vi "2_1_PatchCore_Inference(Image)(Batch).vi"() -> ()   [LabVIEW 2020]
uses:
  PatchCore_AddOn/API/Controls/Heatmap_Config.ctl
  PatchCore_AddOn/API/Controls/ColorMap.ctl
  PatchCore_AddOn/API/Controls/MinMax.ctl
  PatchCore_AddOn/API/Controls/Feature_Scorer_Params.ctl
  PatchCore_AddOn/API/Controls/Gaussian_Blur.ctl
  PatchCore_AddOn/API/Controls/NNPC_Init_Custom_NN_CFG.ctl
  <vilib>/Ngene/Deep Learning Toolkit/Toolkit/NN_Data/API/NN_Dims(C,H,W).ctl
  PatchCore_AddOn/API/Controls/NNPC_Device.ctl
  <vilib>/Ngene/Deep Learning Toolkit/Toolkit/NN_Network/Controls/NN_Device.ctl
  PatchCore_AddOn/API/Controls/NNPC_Trained_Model_Paths.ctl
  PatchCore_AddOn/API/Controls/NN_Paths.ctl
  <vilib>/Utility/miscctls.llb/LVMinMaxIncTypeDef.ctl
  subVIs/Dataset_Reader/Controls/ImRead_PreProcessing_Options.ctl
  PatchCore_AddOn/Low_Level/Controls/Normalization_Type.ctl
  <vilib>/Analysis/baseanly.llb/Mean (DBL).vi
  PatchCore_AddOn/API/NNPC_Predict/NNPC_Predict(Batch).vi
  PatchCore_AddOn/PatchCore_AddOn.lvlib
  <vilib>/ptbypt/NI_PtbyPt.lvlib
  <vilib>/Analysis/NI_AALBase.lvlib
  <vilib>/Ngene/Deep Learning Toolkit/Toolkit/Deep_Learning_Toolkit_by_Ngene.lvlib
panel:
  in  "NNFE PatchCore Paths":T1={"NNFE_Paths"={"CFG"=path "D:/PatchCore/__24_12_11__22_07_40/wrn_50_2_timm_NNFE__24_12_11__22_07_40.cfg", "BIN"=path "D:/PatchCore/__24_12_11__22_07_40/wrn_50_2_timm_NNFE__24_12_11__22_07_40.bin"}, "PatchCore_Paths"={"CFG"=path "D:/PatchCore/__24_12_11__22_07_40/wrn_50_2_timm_Patchcore__24_12_11__22_07_40.cfg", "BIN"=path "D:/PatchCore/__24_12_11__22_07_40/wrn_50_2_timm_MemBank__PS3_RP296_SR0.1_Size16.4k__24_12_11__22_07_40.bin"}}
  in  "Device_Config.":T3={"Device"=enum."GPU", "GPU Id"=0}
  in  "Eval_Stats_File_Path":path=path "D:/PatchCore/__24_12_11__22_07_40/PatchCore_Eval_Stats__24_12_11__22_13_40.cfg"
  in  "NNFE_Custom_CFG":T5={"Input3D_Custom_Dims"={"C"=-1, "H"=-1, "W"=-1}, "mBatch"=8}
  in  "Ground_Truth_Folder_Path":path=path "D:/MVTec/bottle/ground_truth"
  in  "Test_Dataset_Folder_Path":path=path "D:/MVTec/bottle/test"
  in  "Batch_idx":u32 max=74
  in  "Pixel_Thrshld(Custom)":sgl=-1.0 format="%_5g"
  out "Img_Score":sgl=22.713667
  out "Anomaly Detection Results":T7(plugin-control)
  out "Anomaly?":bool
  in  "Stop":bool
  out "Pixel_Thrshld (Eval)":sgl=25.5661
  out "dT_ImRead":dbl=0.02234118052628889 format="%#_4ps"
  out "Image_File_Path":path=path "D:/MVTec/bottle/test/good/000.png"
  out "Pixel_Score(Max)":sgl=27.324837
  out "Pixel_Score(Min)":sgl=2.317538
  out "dT_Predict(Batch)":dbl=0.0410997536842938 format="%#_3ps"
  in  "Feature_Scorer_Params":T8={"Nearest_Neihbours"=1, "Calculate Anomaly Map"=TRUE, "Gaussian_Blur"={"Kernel_Size"=33, "sigma"=4.0}}
  in  "Report_Image_Dims":cluster{"X Resolution":i32, "Y Resolution":i32}={"X Resolution"=224, "Y Resolution"=224}
  in  "Heatmap_Config":T10={"ColorMap_Type"=enum."Jet", "Alpha"=0.4, "Heatmap Range"={"Min"=-1.0, "Max"=-1.0}} {"Heatmap Range"."Min" format="%#_5g"}
  in  "Image_Thrshld(Custom)":sgl=-1.0 format="%_5g"
  out "Image_Thrshld (Eval)":sgl=30.7657
  in  "Image_idx":u32 max=7
  out "Batch Image File Paths":path[](array[path])=[path "D:/MVTec/bottle/test/good/000.png", path "D:/MVTec/bottle/test/good/001.png", path "D:/MVTec/bottle/test/good/002.png", path "D:/MVTec/bottle/test/good/003.png", path "D:/MVTec/bottle/test/good/004.png", path "D:/MVTec/bottle/test/good/005.png", path "D:/MVTec/bottle/test/good/006.png", path "D:/MVTec/bottle/test/good/007.png"]
  out "Anomaly?(Batch)":bool[](array[boolean])
  out "Img_Scores(Batch)":sgl[](array[numeric])=[22.713667, 29.501556, 24.734844, 22.781378, 22.935541, 22.427269, 25.48138, 22.724445]
  out "dT_Predict(perImg)":dbl=0.005137469210536725 format="%#_3ps"
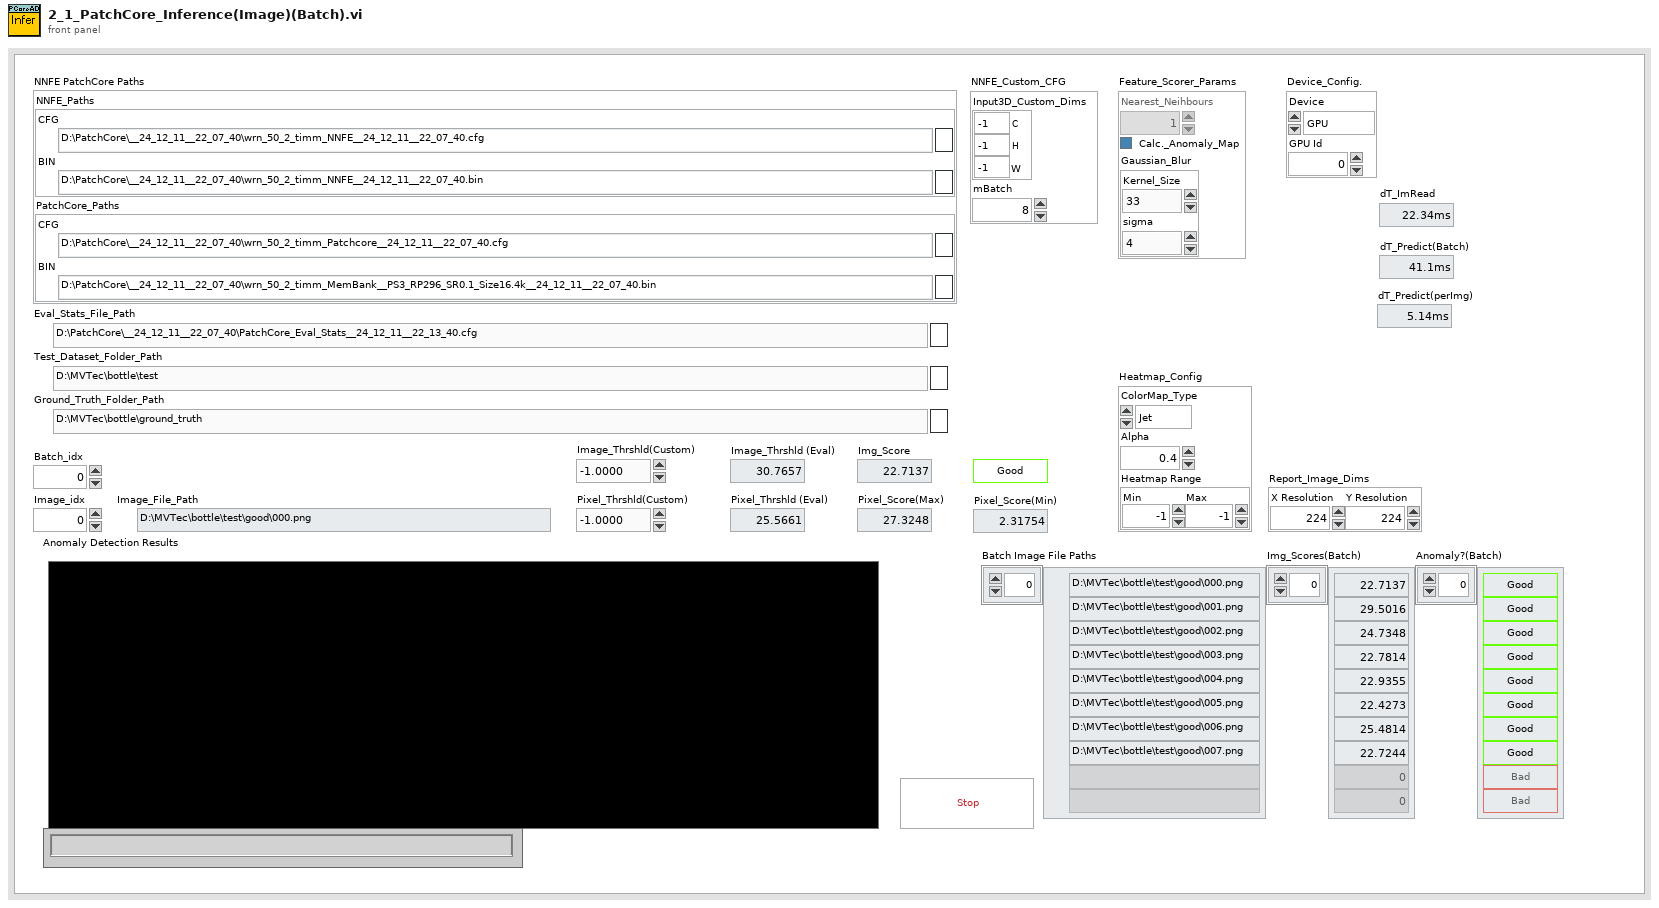
[diagram p1: front panel]
types:
  T1 = typedef "PatchCore_AddOn.lvlib/NNPC_Trained_Model_Paths.ctl" = cluster{"NNFE_Paths":T2, "PatchCore_Paths":T2}
  T2 = typedef "PatchCore_AddOn.lvlib/NN_Paths.ctl" = cluster{"CFG":path, "BIN":path}
  T3 = typedef "PatchCore_AddOn.lvlib/NNPC_Device.ctl" = cluster{"Device":T4, "GPU Id":i32}
  T4 = typedef "Deep_Learning_Toolkit_by_Ngene.lvlib/NN_Device.ctl" = enum16{"CPU", "GPU"}
  T5 = typedef "PatchCore_AddOn.lvlib/NNPC_Init_Custom_NN_CFG.ctl" = cluster{"Input3D_Custom_Dims":T6, "mBatch":i32}
  T6 = typedef "Deep_Learning_Toolkit_by_Ngene.lvlib/NN_Dims(C,H,W).ctl" = cluster{"C":i32, "H":i32, "W":i32}
  T7 = typedef "IMAQ Image.ctl" = refnum<image>
  T8 = typedef "PatchCore_AddOn.lvlib/Feature_Scorer_Params.ctl" = cluster{"Nearest_Neihbours":i32, "Calculate Anomaly Map":bool, "Gaussian_Blur":T9}
  T9 = typedef "PatchCore_AddOn.lvlib/Gaussian_Blur.ctl" = cluster{"Kernel_Size":i32, "sigma":sgl}
  T10 = typedef "PatchCore_AddOn.lvlib/Heatmap_Config.ctl" = cluster{"ColorMap_Type":T11, "Alpha":sgl, "Heatmap Range":T12}
  T11 = typedef "PatchCore_AddOn.lvlib/ColorMap.ctl" = enum16{"Jet", "Perula", "Inferno", "Plasma", "Viridis"}
  T12 = typedef "PatchCore_AddOn.lvlib/MinMax.ctl" = cluster{"Min":sgl, "Max":sgl}
  T13 = typedef "LVMinMaxIncTypeDef.ctl" = cluster{"Minimum":dbl, "Maximum":dbl, "Increment":dbl}
  T14 = typedef "PatchCore_AddOn.lvlib/NNPC_Instance.ctl" = cluster{"Dataset_Stats":T15, "NN":T17, "Device_Config.":T3, "PatchCore_Init_CFG":T32, "Coreset Params":T34, "MemBank_Data":T36}
  T15 = typedef "PatchCore_AddOn.lvlib/NNPC_DS_Stats.ctl" = cluster{"means":T16, "vars":T16, "DS_Size":i32}
  T16 = typedef "PatchCore_AddOn.lvlib/Image_Stats_RGB.ctl" = cluster{"R":sgl, "G":sgl, "B":sgl}
  T17 = typedef "Deep_Learning_Toolkit_by_Ngene.lvlib/NN.ctl" = cluster{"Name":string, "No of Layers":i32, "mBatch":i32, "Layers":T18[], "Dimty":T19, "Dims_In":T6, "Dims_Out":T6, "Working_Dir":path, "Train?":bool, "Train_Params":T20, "LR_Update_Policy":T23, "Session Data":T25, "Ground_truth":T26, "NNg_hdls":T27, "NN_Device":T4, "GPU Id":i32, "Labels":string[], "Receptive Field":T28[], "Loss_Type":T29, "Loss_Cfg_Prms":variant, "NNG_WS":T30}
  T18 = typedef "Deep_Learning_Toolkit_by_Ngene.lvlib/NN_Layer_ref.ctl" = refnum<data-value>
  T19 = typedef "Deep_Learning_Toolkit_by_Ngene.lvlib/NN_In_Out_Dim-ty.ctl" = enum8{"In1D_Out1D", "In3D_Out1D", "In3D_Out3D", "In3D_OutBBox"}
  T20 = typedef "Deep_Learning_Toolkit_by_Ngene.lvlib/NN_Train_Params.ctl" = cluster{"Optimizer":T21, "Beta_1":sgl, "Beta_2":sgl, "Weight Decay(L1)":sgl, "Weight Decay(L2)":sgl, "Data_Sampling":T22}
  T21 = typedef "Deep_Learning_Toolkit_by_Ngene.lvlib/NN_Train_Optimizer.ctl" = enum16{"SGD", "Adam", "Adagrad", "Adadelta", "RMSProp", "Nesterov"}
  T22 = typedef "Deep_Learning_Toolkit_by_Ngene.lvlib/NN_Train_Data_Sampling.ctl" = enum16{"Random", "Sequential"}
  T23 = typedef "Deep_Learning_Toolkit_by_Ngene.lvlib/NN_LR_Policy_Cfg.ctl" = cluster{"Policy_Type":T24, "LR0":dbl, "k":sgl, "WarmUp_Policy":enum16{"Step", "Ramp"}, "WarmUp_Iter":i32, "WarmUp_Ratio":sgl}
  T24 = typedef "Deep_Learning_Toolkit_by_Ngene.lvlib/NN_LR_Policy_Type.ctl" = enum16{"Manual", "Step", "Exp", "1/t"}
  T25 = typedef "Deep_Learning_Toolkit_by_Ngene.lvlib/NN_Train_Session_Data.ctl" = cluster{"Epochs":sgl, "Tot_Iter":i32, "LR":sgl, "LR_iter":i32}
  T26 = typedef "Deep_Learning_Toolkit_by_Ngene.lvlib/NN_Ground_truth.ctl" = cluster{"Y":variant}
  T27 = typedef "Deep_Learning_Toolkit_by_Ngene.lvlib/nng_cuda_handles.ctl" = cluster{"cudnn":u64, "cublas":u64, "stream":u64, "curand":u64}
  T28 = typedef "Deep_Learning_Toolkit_by_Ngene.lvlib/NN_Dims(V,H).ctl" = cluster{"V":i32, "H":i32}
  T29 = typedef "Deep_Learning_Toolkit_by_Ngene.lvlib/NN_Loss_Type.ctl" = enum16{"None", "MSE", "CrossEntropy", "YOLO_v2", "YOLO_v4"}
  T30 = typedef "Deep_Learning_Toolkit_by_Ngene.lvlib/NNG_WS.ctl" = cluster{"NNG_WS_Mem":T31, "Max_WS_Size":i64}
  T31 = typedef "Deep_Learning_Toolkit_by_Ngene.lvlib/NNg_WS_Mem_DVR.ctl" = refnum<data-value>
  T32 = typedef "PatchCore_AddOn.lvlib/NNPC_Init_CFG.ctl" = cluster{"BackBone":T33, "Out_Layers_Names":string[], "Patch_Size":u32}
  T33 = typedef "PatchCore_AddOn.lvlib/NNPC_BackBone_Selector.ctl" = enum16{"WRN_50_2_L2L3"}
  T34 = typedef "PatchCore_AddOn.lvlib/NNPC_Coreset_Params.ctl" = cluster{"Name":string, "Sampling_Ratio":sgl, "Startd_idx":i32, "Random_Proj?":bool, "Rnd. Proj. Params":T35}
  T35 = typedef "PatchCore_AddOn.lvlib/NNPC_Random_Projection_CFG.ctl" = cluster{"Proj._Dim.":i32, "Epsilon":sgl, "Seed":i32}
  T36 = typedef "PatchCore_AddOn.lvlib/MemBank_and_Norm_Variants.ctl" = cluster{"MemBank":variant, "MemBank Norm":variant}
  T37 = typedef "PatchCore_AddOn.lvlib/Eval_Results.ctl" = cluster{"Scores(Good)":T12, "Scores(Bad)":T12, "F1_Max":sgl, "Thrshld(F1_Max)":sgl, "IoU_Max":sgl, "Thrshld(IoU_Max)":sgl, "AUROC":sgl, "Prec.(F1_Max)":sgl, "Recall(F1_Max)":sgl, "FPR(F1_Max)":sgl, "FNR(F1_Max)":sgl}
  T38 = typedef "ImRead_PreProcessing_Options.ctl" = cluster{"Image Type":T39, "Normalization Type":T40, "Interpolation Type":u32}
  T39 = typedef "Image Type" = u32
  T40 = typedef "PatchCore_AddOn.lvlib/Normalization_Type.ctl" = enum16{"Standardize(DS_Stats)", "Standardize(Image_Stats)"}
  T41 = typedef "PatchCore_AddOn.lvlib/Anomaly_Detection_Results_Imgs.ctl" = cluster{"Image":T7, "Ground Truth":T7, "Predicted Heat Map":T7, "Predicted Mask":T7, "Segmentation":T7}
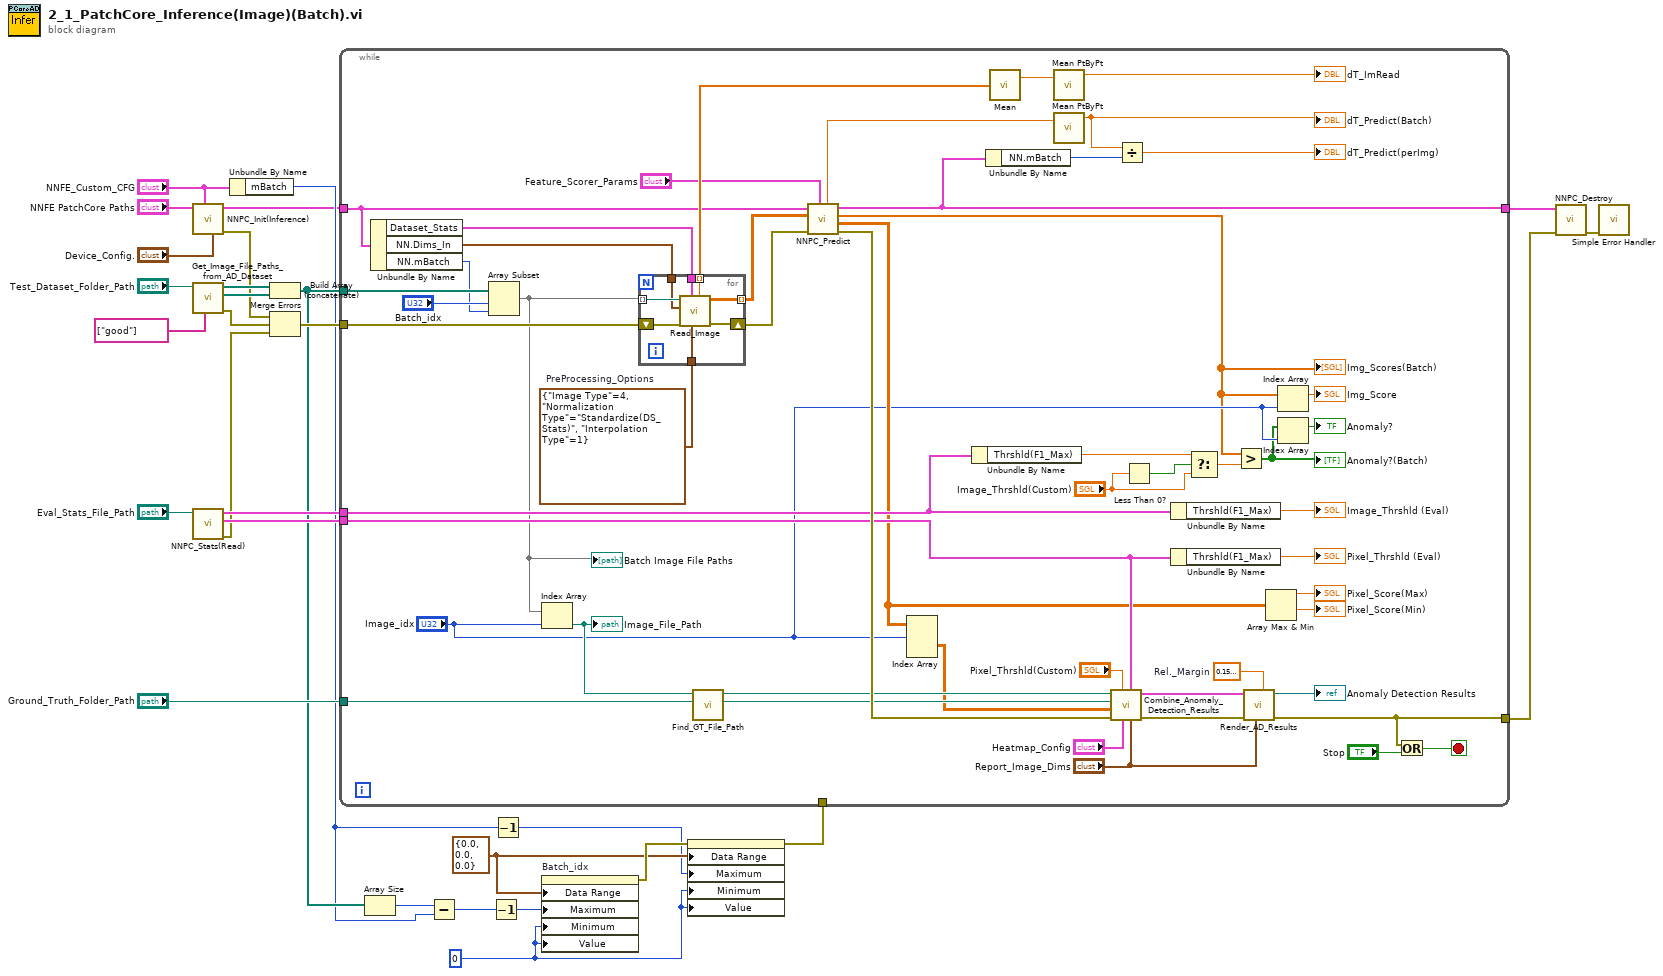
[diagram p0: block diagram]
diagram:
  w11 = T13 {"Minimum"=0.0, "Maximum"=0.0, "Increment"=0.0} ("Data Entry Limits")
  w9 = u32 0 ("Data Entry Limits:Minimum")
  n1 = call "NNPC_Init(Inference).vi"("Device_Config."="Device_Config.", "NNFE_Custom_CFG"="NNFE_Custom_CFG", "NNFE PatchCore Paths"="NNFE PatchCore Paths") -> ("error out"=w2:errorcluster, "PCore_Instance out"=w5:T14)  [unwired: 7 in]
  n2 = call "Get_Image_File_Paths_from_AD_Dataset.vi"("Good Folder Names"=string[] ["good"] ("Good Folder Name"), "Dataset Folder"="Test_Dataset_Folder_Path") -> ("error out"=w18:errorcluster, "Bad Dataset Files"=w14:path[], "Good Dataset Files"=w13:path[])  [unwired: 7 in]
  n3 = call "NNPC_Stats(Read).vi"("CFG file path"="Eval_Stats_File_Path") -> ("error out"=w22:errorcluster, "Pixel Results"=w23:T37, "Image Results"=w24:T37)  [unwired: 8 in]
  n4 = Unbundle By Name("NNFE_Custom_CFG") -> ("mBatch"=w7:i32)
  n5 = Build Array (concatenate)(w13, w14) -> (w19:path[])
  n6 = Merge Errors(w2, w18, w22) -> (w25:errorcluster)
  n7 = Array Size(array=w19) -> (size(s)=w29:i32)
  n8 = Subtract(x=w29, y=w7) -> (x-y=w8:i32)
  n9 = Decrement(x=w8) -> (x-1=w28:i32)
  n10 = Decrement(x=w7) -> (x-1=w10:i32)
  n11 = property on="Batch_idx" class="DigNum (strict)"("Data Range"=w11, "Maximum"=w28, "Minimum"=w9, "Value"=w9) -> (error out=w12:errorcluster)  [unwired: 2 in, 1 out]
  n12 = property on="Image_idx" class="DigNum (strict)"(error in=w12, "Data Range"=w11, "Maximum"=w10, "Minimum"=w9, "Value"=w9) -> (error out=w6:errorcluster)  [unwired: 1 in, 1 out]
  n13 = while {
    tunnel: w19 -> [w81]
    tunnel: w5 -> [w61]
    tunnel: [w33] -> w16
    tunnel: w24 -> [w55]
    tunnel: w23 -> [w54]
    tunnel: w25 -> [w80]
    tunnel: [w30] -> w17
    tunnel: "Ground_Truth_Folder_Path" -> [w64]
    tunnel: w6 -> [_]
    stop <- w31 stop-if-true
    w73 = sgl 0.15  # Rel._Margin
    w50 = T38 {"Image Type"=4, "Normalization Type"=enum."Standardize(DS_Stats)", "Interpolation Type"=1}  # PreProcessing_Options
    n14 = Unbundle By Name(w61) -> ("Dataset_Stats"=w52:T15, "NN.Dims_In"=w51:T6, "NN.mBatch"=w46:i32)
    n15 = Array Subset(array=w81, index="Batch_idx", length=w46) -> (w47:path[])
    "Batch Image File Paths" <- w47
    n16 = Index Array(array=w47, index="Image_idx") -> (element=w48:path)
    "Image_File_Path" <- w48
    n17 = for {
      tunnel: [w88] -> w67 mode=indexing
      tunnel: w47 -> [w87] mode=indexing
      tunnel: [w86] -> w38 mode=indexing
      tunnel: w52 -> [w84]
      tunnel: w51 -> [w83]
      tunnel: w50 -> [w82]
      shift-right: [w85] -> w53
      shift-left: w80 -> [w89]
      n18 = call "Read_Image.vi"("PreProcessing_Options"=w82, "Dataset_Stats"=w84, "error in"=w89, "Target_Dims"=w83, "Img Path"=w87) -> ("error out"=w85:errorcluster, "Image Out"=w86:sgl[][][], "dT_Img_Read"=w88:dbl)  [unwired: 4 in]
    }
    n19 = call "Find_GT_File_Path.vi"("GT Mask Folder Path"=w64, "Image File Path"=w48) -> ("GT File Path"=w65:path, "Image File Path out"=w66:path)  [unwired: 8 in]
    n20 = call-poly "NNPC_Predict.vi"("Feature Scorer Params"="Feature_Scorer_Params", "error in (no error)"=w53, "Image(Batch)"=w38, "PCore_Instance in"=w61) -> ("error out"=w78:errorcluster, "anomaly maps"=w44:sgl[][][], "pred scores"=w39:sgl[], "PCore_Instance out"=w33:T14, "dT_Predict"=w60:dbl)  [unwired: 3 in]
    "Img_Scores(Batch)" <- w39
    n21 = Index Array(array=w44, index (dim 0)="Image_idx") -> (element=w45:sgl[][])  [unwired: 2 in]
    n22 = Unbundle By Name(w55) -> ("Thrshld(F1_Max)"=w69:sgl)
    n23 = Unbundle By Name(w33) -> ("NN.mBatch"=w32:i32)
    n24 = call-poly <vilib>:"Mean.vi"("X"=w67) -> ("mean"=w37:dbl)  [unwired: 1 out]
    n25 = call <vilib>:"Mean PtByPt.vi"("x"=w37) -> ("mean"=→"dT_ImRead":dbl)  [unwired: 3 in, 1 out]
    n26 = call <vilib>:"Mean PtByPt.vi"("x"=w60) -> ("mean"=w35:dbl)  [unwired: 3 in, 1 out]
    "dT_Predict(Batch)" <- w35
    n27 = call "Combine_Anomaly_Detection_Results.vi"("Infrnc Dims"="Report_Image_Dims", "Pixel Results"=w54, "Heatmap Config"="Heatmap_Config", "Pixel Anomaly Thrshld"="Pixel_Thrshld(Custom)", "error in"=w78, "Anomaly Map"=w45, "Gt File Path"=w65, "Img File Path"=w66) -> ("error out"=w77:errorcluster, "Anomaly Detection Rresults"=w76:T41)  [unwired: 1 in, 1 out]
    n28 = Divide(x=w35, y=w32) -> (x/y=→"dT_Predict(perImg)":dbl)
    n29 = Less Than 0?(x="Image_Thrshld(Custom)") -> (x < 0?=w71:bool)
    n30 = Unbundle By Name(w55) -> ("Thrshld(F1_Max)"=→"Image_Thrshld (Eval)":sgl)
    n31 = Unbundle By Name(w54) -> ("Thrshld(F1_Max)"=→"Pixel_Thrshld (Eval)":sgl)
    n32 = Select(t=w69, s=w71, f="Image_Thrshld(Custom)") -> (s? t:f=w68:sgl)
    n33 = Greater?(x=w39, y=w68) -> (0:w40:bool[])
    "Anomaly?(Batch)" <- w40
    n34 = call "Render_AD_Results.vi"("Rel._Margin"=w73, "Image_Dims"="Report_Image_Dims", "error in"=w77, "Anomaly Detection Rresults"=w76) -> ("error out"=w30:errorcluster, "Anomaly Detection Results"=→"Anomaly Detection Results":T7)  [unwired: 6 in]
    n35 = Array Max & Min(array=w44) -> (max value=→"Pixel_Score(Max)":sgl, min value=→"Pixel_Score(Min)":sgl)  [unwired: 2 out]
    n36 = Index Array(array=w39, index="Image_idx") -> (element=→"Img_Score":sgl)
    n37 = Index Array(array=w40, index="Image_idx") -> (element=→"Anomaly?":bool)
    n38 = Or(x=w30, y="Stop") -> (x .or. y?=w31:bool)
  }
  n39 = call "NNPC_Destroy.vi"("error in"=w17, "PCore_Instance in"=w16) -> ("error out"=w15:errorcluster)  [unwired: 9 in]
  n40 = call <vilib>:"Simple Error Handler.vi"("error in (no error)"=w15) -> ()  [unwired: 4 in, 5 out]
